vi "FIFO Test.vi"() -> ()   [LabVIEW 2018]
uses:
  <vilib>/LabVIEW Targets/FPGA/cRIO/shared/nicrio_ModuleControls/nicrio_cRIO-9237_DataRatesRing.ctl
  <vilib>/FPGAPlugInAG/cRIO-9074/niLvFpga_Open_cRIO-9074.vi
  <vilib>/Utility/error.llb/Error Cluster From Error Code.vi
  <vilib>/rvi/errors/niLvFpgaAdjustHostInterfaceError.vi
  <vilib>/FPGAPlugInAG/cRIO-9074/niLvFpga_Close_cRIO-9074.vi
  <vilib>/rvi/interface/nirviOpenFPGA/nirviOpenFPGA.xnode
  FPGA Bitfiles/NewCompressorRig_FPGATarget_FPGAMain_dxecnm0rUT0.lvbitx
  FPGA/FPGA Main.vi
  <vilib>/rvi/interface/nirviReadWriteControl/nirviReadWriteControl.xnode
  <vilib>/rvi/interface/nirviMethod/nirviMethod.xnode
  <vilib>/rvi/interface/nirviCloseFPGA/nirviCloseFPGA.xnode
  NiFpgaLv.dll
  <vilib>/rvi/errors/niLvFpgaMergeErrorWithErrorCode.vi
  <vilib>/FPGAPlugInAG/cRIO-9074/niLvFpga_ReadFifo_cRIO-9074.vi
  <vilib>/FPGAPlugInAG/cRIO-9074/niLvFpga_StartFifo_cRIO-9074.vi
  <vilib>/FPGAPlugInAG/cRIO-9074/niLvFpga_StopFifo_cRIO-9074.vi
panel:
  out "Max remainder":u32
  out "appended array":errorcluster[](array[cluster])
  out "loop period (usec)":u32
  in  "Stop":bool
  out "subarray":sgl[](array[numeric])
  out "error out":errorcluster
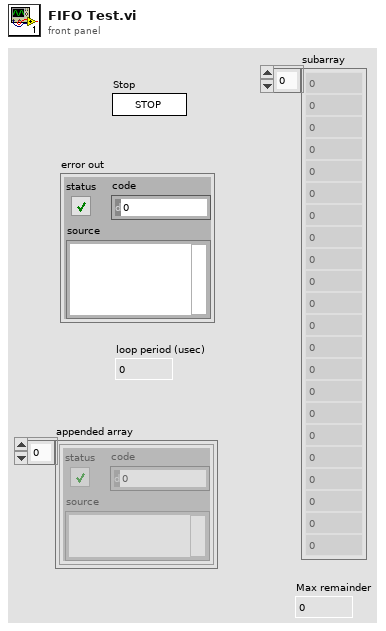
[diagram p1: front panel]
types:
  T1 = typedef "nicrio_cRIO-9237_DataRatesRing.ctl" = u8
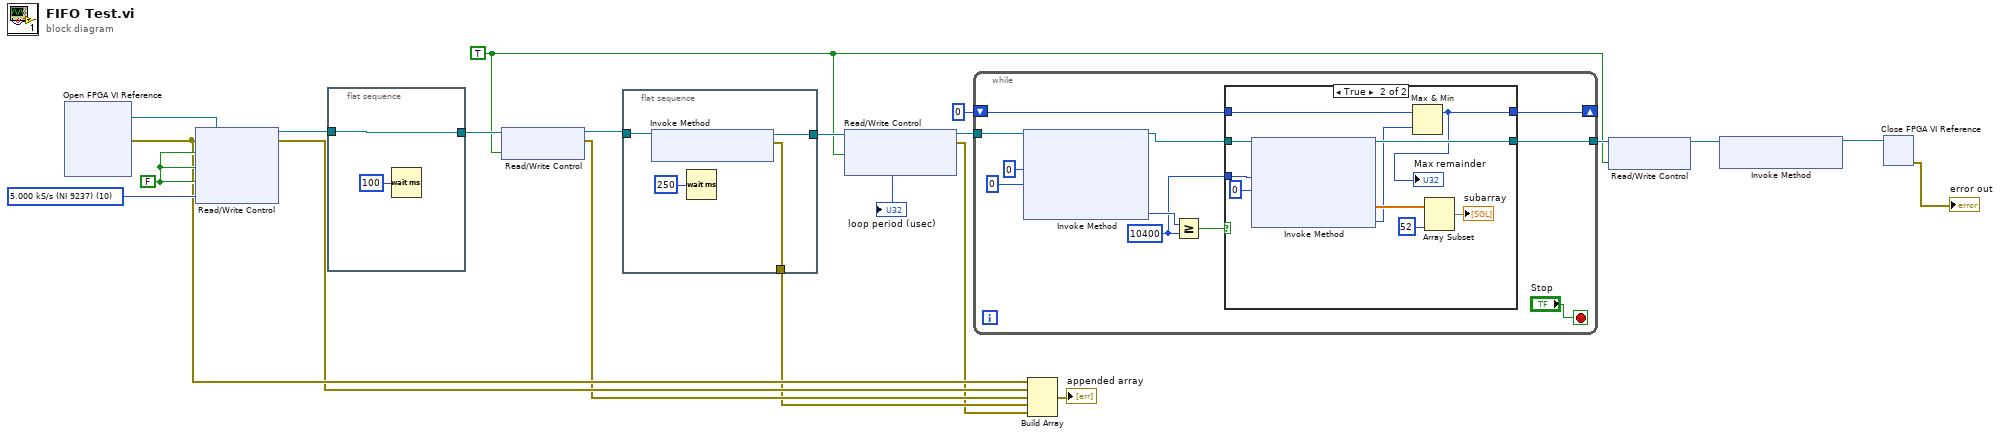
[diagram p0: block diagram]
diagram:
  w12 = TRUE ("Start acquire")
  w19 = T1 10 items=["50.000 kS/s (NI 9237)"=1, "25.000 kS/s (NI 9237)"=2, "16.667 kS/s (NI 9237)"=3, "12.500 kS/s (NI 9237)"=4, "10.000 kS/s (NI 9237)"=5, "8.333 kS/s (NI 9237)"=6, "7.143 kS/s (NI 9237)"=7, "6.250 kS/s (NI 9237)"=8, "5.556 kS/s (NI 9237)"=9, "5.000 kS/s (NI 9237)"=10, "4.545 kS/s (NI 9237)"=11, "4.167 kS/s (NI 9237)"=12, "3.846 kS/s (NI 9237)"=13, "3.571 kS/s (NI 9237)"=14, "3.333 kS/s (NI 9237)"=15, "3.125 kS/s (NI 9237)"=16, "2.941 kS/s (NI 9237)"=17, "2.778 kS/s (NI 9237)"=18, "2.632 kS/s (NI 9237)"=19, "2.500 kS/s (NI 9237)"=20, "2.381 kS/s (NI 9237)"=21, "2.273 kS/s (NI 9237)"=22, "2.174 kS/s (NI 9237)"=23, "2.083 kS/s (NI 9237)"=24, "2.000 kS/s (NI 9237)"=25, "1.923 kS/s (NI 9237)"=26, "1.852 kS/s (NI 9237)"=27, "1.786 kS/s (NI 9237)"=28, "1.724 kS/s (NI 9237)"=29, "1.667 kS/s (NI 9237)"=30, "1.613 kS/s (NI 9237)"=31] ("Data Rate")
  w20 = FALSE ("Start acquire")
  n1 = xnode "Open FPGA VI Reference"() -> ("FPGA VI Reference Out"=w21:refnum<k20>, "error out"=w7:errorcluster)  [unwired: 2 in]
  n2 = xnode "Read/Write Control"("FPGA VI Reference In"=w21, "error in"=w7, "Stop acquire"=w20, "Exit"=w20, "Start acquire"=w20, "Data Rate"=w19) -> ("FPGA VI Reference Out"=w18:refnum<k20>, "error out"=w6:errorcluster)
  n3 = flat-sequence {
    tunnel: [w23] -> w17
    tunnel: w18 -> [w23]
    frame #0 {
      n4 = Wait (ms)(milliseconds to wait=u32 100) -> ()  [unwired: 1 out]
    }
  }
  n5 = xnode "Read/Write Control"("FPGA VI Reference In"=w17, "Start acquire"=w12) -> ("FPGA VI Reference Out"=w16:refnum<k20>, "error out"=w5:errorcluster)  [unwired: 1 in]
  n6 = flat-sequence {
    tunnel: [w25] -> w15
    tunnel: w16 -> [w26]
    tunnel: [w24] -> w4
    frame #0 {
      n7 = xnode "Invoke Method"("FPGA VI Reference In"=w26) -> ("FPGA VI Reference Out"=w25:refnum<k20>, "error out"=w24:errorcluster)  [unwired: 1 in]
      n8 = Wait (ms)(milliseconds to wait=u32 250) -> ()  [unwired: 1 out]
    }
  }
  n9 = xnode "Read/Write Control"("FPGA VI Reference In"=w15, "Enable FIFO"=w12) -> ("FPGA VI Reference Out"=w14:refnum<k20>, "error out"=w3:errorcluster, "loop period (usec)"=→"loop period (usec)":u32)  [unwired: 1 in]
  n10 = while {
    tunnel: w14 -> [w38]
    tunnel: [w30] -> w13
    shift-right: [w29] -> _
    shift-left: u32 0 -> [w28]
    stop <- "Stop" stop-if-true
    w33 = u32 10400 ("y")
    n11 = xnode "Invoke Method"("FPGA VI Reference In"=w38, "Number of Elements"=u32 0, "Timeout (ms)"=0) -> ("FPGA VI Reference Out"=w32:refnum<k20>, "Elements Remaining"=w37:u32)  [unwired: 1 in, 2 out]
    n12 = Greater Or Equal?(x=w37, y=w33) -> (x >= y?=w36:bool)
    n13 = case shown="True" w36 {
      tunnel: w33 -> [_ w49]
      tunnel: w32 -> [w40 w48]
      tunnel: [w40 w44] -> w30
      tunnel: w28 -> [w39 w43]
      tunnel: [w39 w41] -> w29
      frame False {
      }
      frame True {
        n14 = xnode "Invoke Method"("FPGA VI Reference In"=w48, "Number of Elements"=w49, "Timeout (ms)"=0) -> ("FPGA VI Reference Out"=w44:refnum<k20>, "Data"=w47:sgl[], "Elements Remaining"=w42:u32)  [unwired: 1 in, 1 out]
        n15 = Max & Min(x=w43, y=w42) -> (max(x,y)=w41:u32)  [unwired: 1 out]
        "Max remainder" <- w41
        n16 = Array Subset(array=w47, length=52) -> (→"subarray":sgl[])  [unwired: 1 in]
      }
    }
  }
  n17 = Build Array(w7, w6, w5, w4, w3) -> (→"appended array":errorcluster[])
  n18 = xnode "Read/Write Control"("FPGA VI Reference In"=w13, "Stop acquire"=w12) -> ("FPGA VI Reference Out"=w11:refnum<k20>)  [unwired: 1 in, 1 out]
  n19 = xnode "Invoke Method"("FPGA VI Reference In"=w11) -> ("FPGA VI Reference Out"=w10:refnum<k20>)  [unwired: 1 in, 1 out]
  n20 = xnode "Close FPGA VI Reference"("FPGA VI Reference In"=w10) -> ("error out"=→"error out":errorcluster)  [unwired: 1 in]
